vi "Double Acq test RT.vi"() -> ()   [LabVIEW 2014]
uses:
  <vilib>/Platform/TimedLoop/XDataNode/timing_clust.ctl
  <vilib>/Platform/TimedLoop/XDataNode/nitl_modes.ctl
  <vilib>/Platform/TimedLoop/XDataNode/wakeup.ctl
  <vilib>/FPGAPlugInAG/sbRIO-9636/niLvFpga_Open_sbRIO-9636.vi
  <vilib>/rvi/interface/common/dynamic/niFpgaDynamicAddResources.vi
  <vilib>/rvi/interface/common/niFpgaWaitOnOcc.vi
  <vilib>/Utility/error.llb/Error Cluster From Error Code.vi
  <vilib>/FPGAPlugInAG/Dynamic/niLvFpga_Run_Dynamic.vi
  <vilib>/rvi/errors/niLvFpgaAdjustHostInterfaceError.vi
  <vilib>/FPGAPlugInAG/Dynamic/niLvFpga_Abort_Dynamic.vi
  <vilib>/FPGAPlugInAG/Dynamic/niLvFpga_Close_Dynamic.vi
  <vilib>/rvi/interface/nirviOpenFPGA/nirviOpenFPGA.xnode
  FPGA Bitfiles/LaserDistanceSen_FPGATarget_DoubleAcquisitio_6KO4bY+0XGM.lvbitx
  FPGA Target/Test VIs/Double Acquisition (Mod-Sign) test.vi
  <vilib>/rvi/interface/nirviMethod/nirviMethod.xnode
  <vilib>/Platform/TimedLoop/XDataNode/XDataNode.xnode
  <vilib>/rvi/interface/nirviReadWriteControl/nirviReadWriteControl.xnode
  <vilib>/rvi/interface/nirviCloseFPGA/nirviCloseFPGA.xnode
  <vilib>/rvi/interface/Simulation/niFpgaSimulationCallBeginRW.vi
  <vilib>/FPGAPlugInAG/Dynamic/niLvFpga_ConfigureFifo_Dynamic.vi
  <vilib>/rvi/errors/niLvFpgaMergeErrorWithErrorCode.vi
  <vilib>/FPGAPlugInAG/Dynamic/niLvFpga_StartFifo_Dynamic.vi
  <vilib>/FPGAPlugInAG/Dynamic/niLvFpga_ReadFifo_Dynamic.vi
  <vilib>/Platform/TimedLoop/XDataNode/XDNodeRunTimeDep.lvlib
  NiFpgaLv.dll
panel:
  out "Modulation Signal":dbl[](graph)
  out "Signal":dbl[](graph)
  in  "stop":bool
  in  "Snapshot":bool
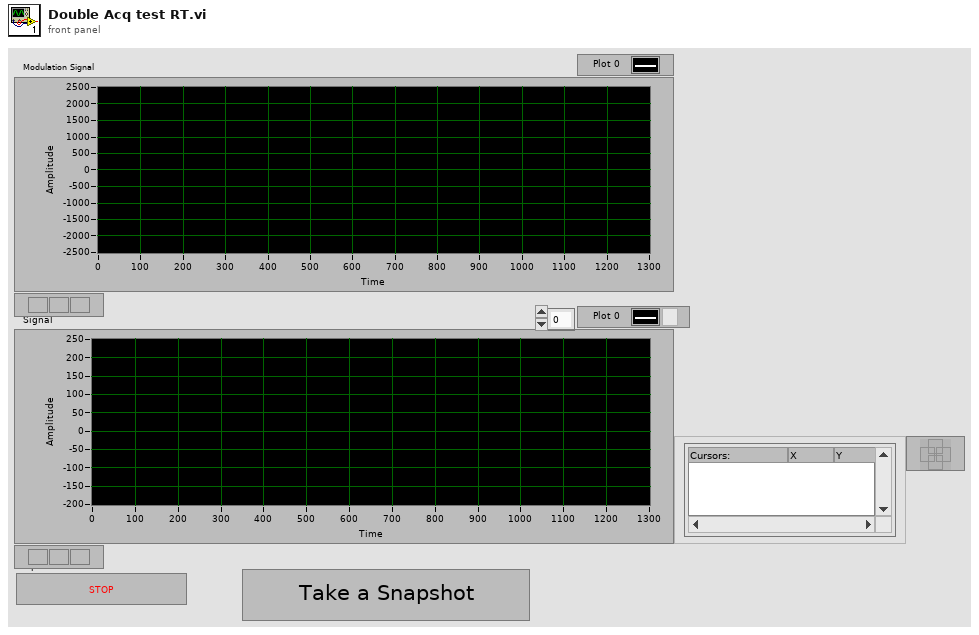
[diagram p1: front panel]
types:
  T1 = typedef "XDNodeRunTimeDep.lvlib/timing_clust.ctl" = cluster{"Expected End [f-1]":u64, "Actual End [f-1]":u64, "Finished Late? [f-1]":bool, "Expected End [i-1]":u64, "Actual End [i-1]":u64, "Finished Late? [i-1]":bool, "Expected Start [i]":u64, "Actual Start [i]":u64, "Expected Start [f]":u64, "Actual Start [f]":u64, "Source Name":string, "Structure Name":string, "Period":i64, "Deadline":i64, "Offset":i64, "Start":i64, "Priority":i32, "Timeout":i32, "Mode":T2, "Wakeup Reason":T3, "Error":errorcluster, "Source Type":string, "Secondary Source Type":string, "Global End Time":u64, "Global Start Time":u64, "Frame Duration":u64, "Iteration Duration":u64, "Assigned CPU":i32, "I/O Scan Engine Mode":u32}
  T2 = typedef "XDNodeRunTimeDep.lvlib/nitl_modes.ctl" = enum32{"No Change", "Process missed periods, maintain original phase", "Discard missed periods, maintain original phase", "Process missed periods, ignore original phase", "Discard missed periods, ignore original phase"}
  T3 = typedef "XDNodeRunTimeDep.lvlib/wakeup.ctl" = enum32{"Normal", "Aborted", "Asynchronous wakeup", "Timing source error", "Timed loop error", "Timeout"}
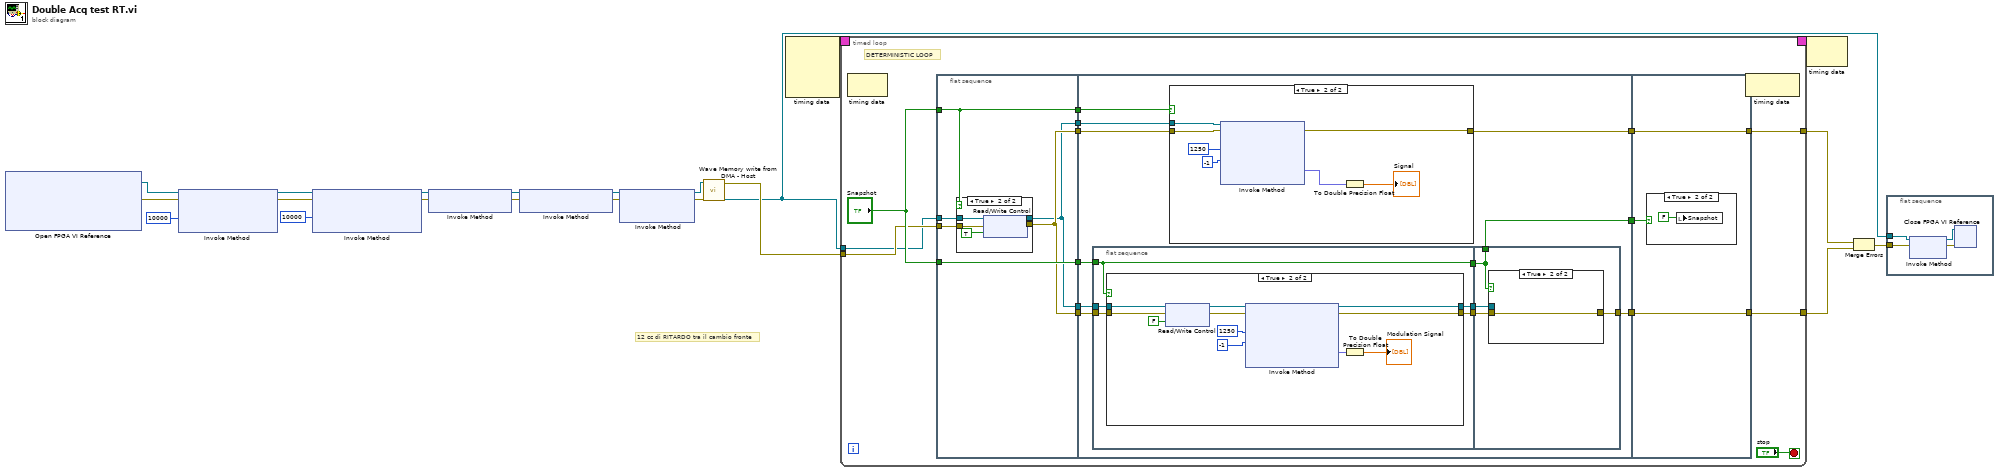
[diagram p0: block diagram]
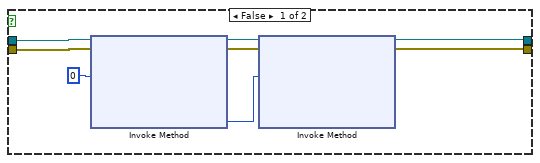
[diagram p3: hidden frame]
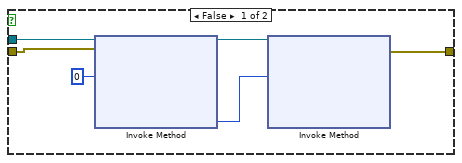
[diagram p5: hidden frame]
diagram:
  # "12 cc di RITARDO tra il cambio fronte"
  n1 = xnode "Open FPGA VI Reference"() -> ("FPGA VI Reference Out"=w8:refnum<k20>, "error out"=w9:errorcluster)  [unwired: 2 in]
  n2 = xnode "Invoke Method"("FPGA VI Reference In"=w8, "error in"=w9, "Requested Depth"=u32 10000) -> ("FPGA VI Reference Out"=w19:refnum<k20>, "error out"=w18:errorcluster)  [unwired: 1 out]
  n3 = xnode "Invoke Method"("FPGA VI Reference In"=w19, "error in"=w18, "Requested Depth"=u32 10000) -> ("FPGA VI Reference Out"=w6:refnum<k20>, "error out"=w7:errorcluster)  [unwired: 1 out]
  n4 = xnode "Invoke Method"("FPGA VI Reference In"=w6, "error in"=w7) -> ("FPGA VI Reference Out"=w15:refnum<k20>, "error out"=w14:errorcluster)
  n5 = xnode "Invoke Method"("FPGA VI Reference In"=w15, "error in"=w14) -> ("FPGA VI Reference Out"=w4:refnum<k20>, "error out"=w5:errorcluster)
  n6 = xnode "Invoke Method"("FPGA VI Reference In"=w4, "error in"=w5) -> ("FPGA VI Reference Out"=w12:refnum<k20>, "error out"=w11:errorcluster)  [unwired: 1 in]
  n7 = call "Wave Memory write from DMA - Host.vi"("error in"=w11, "FPGA VI Reference In"=w12) -> ("FPGA VI Reference Out"=w1:refnum<k20>, "error out"=w3:errorcluster)  [unwired: 7 in, 1 out]
  n8 = node-c288() -> (w21:T1)  [unwired: 4 in]
  n9 = timed-loop {
    tunnel: w1 -> [w32]
    tunnel: w3 -> [w33]
    tunnel: [w35] -> w2
    tunnel: [w36] -> w10
    timing: w21 -> [_]
    timing-out: [_] -> w20
    stop <- "stop" stop-if-true
    # "DETERMINISTIC LOOP"
    n10 = node-c288() -> ()  [unwired: 1 in, 1 out]
    n11 = flat-sequence {
      tunnel: w32 -> [w41]
      tunnel: w33 -> [w42]
      tunnel: "Snapshot" -> [w39]
      tunnel: "Snapshot" -> [w44]
      tunnel: [w43] -> w31
      tunnel: [w44] -> w30
      tunnel: [w39] -> w29
      tunnel: [w43] -> w28
      tunnel: [w40] -> w27
      tunnel: [w40] -> w26
      tunnel: w31 -> [w59]
      tunnel: w30 -> [w52]
      tunnel: w29 -> [w56]
      tunnel: w28 -> [w55]
      tunnel: w27 -> [w54]
      tunnel: w26 -> [w60]
      tunnel: [w58] -> w25
      tunnel: [w57] -> w24
      tunnel: [w53] -> w23
      tunnel: [w108] -> w35
      tunnel: [w109] -> w36
      tunnel: w25 -> [w109]
      tunnel: w24 -> [w108]
      tunnel: w23 -> [w107]
      frame #0 {
        n12 = case shown="True" w39 {
          tunnel: [w45 w50] -> w43
          tunnel: w42 -> [w45 w49]
          tunnel: w41 -> [w46 w48]
          tunnel: [w46 w47] -> w40
          frame False {
          }
          frame True {
            n13 = xnode "Read/Write Control"("FPGA VI Reference In"=w48, "error in"=w49, "Snapshot"=TRUE ("snapshot")) -> ("FPGA VI Reference Out"=w47:refnum<k20>, "error out"=w50:errorcluster)
          }
        }
      }
      frame #1 {
        n14 = flat-sequence {
          tunnel: w60 -> [w68]
          tunnel: w59 -> [w67]
          tunnel: w52 -> [w64]
          tunnel: [w66] -> w63
          tunnel: [w65] -> w62
          tunnel: [w64] -> w61
          tunnel: [w89] -> w57
          tunnel: w63 -> [w91]
          tunnel: w62 -> [w90]
          tunnel: w61 -> [w88]
          tunnel: [w88] -> w53
          frame #0 {
            n15 = case shown="True" w64 {
              tunnel: w68 -> [w75 w78]
              tunnel: w67 -> [w73 w80]
              tunnel: [w72 w85] -> w65
              tunnel: [w69 w84] -> w66
              frame False {
                n16 = xnode "Invoke Method"("FPGA VI Reference In"=w75, "error in"=w73, "Number of Elements"=u32 0) -> ("FPGA VI Reference Out"=w71:refnum<k20>, "error out"=w70:errorcluster, "Elements Remaining"=w74:u32)  [unwired: 1 in, 1 out]
                n17 = xnode "Invoke Method"("FPGA VI Reference In"=w71, "error in"=w70, "Number of Elements"=w74) -> ("FPGA VI Reference Out"=w69:refnum<k20>, "error out"=w72:errorcluster)  [unwired: 1 in, 2 out]
              }
              frame True {
                n18 = xnode "Read/Write Control"("FPGA VI Reference In"=w78, "error in"=w80, "Snapshot"=FALSE ("snapshot")) -> ("FPGA VI Reference Out"=w77:refnum<k20>, "error out"=w79:errorcluster)
                n19 = xnode "Invoke Method"("FPGA VI Reference In"=w77, "error in"=w79, "Number of Elements"=u32 1250, "Timeout (ms)"=-1) -> ("FPGA VI Reference Out"=w84:refnum<k20>, "error out"=w85:errorcluster, "Data"=w83:fxp<+/-,12,12>[])  [unwired: 1 out]
                n20 = To Double Precision Float(number=w83) -> (double precision float=→"Modulation Signal":dbl[])
              }
            }
          }
          frame #1 {
            n21 = case shown="True" w88 {
              tunnel: [w92 w93] -> w89
              tunnel: w91 -> [_ _]
              tunnel: w90 -> [w92 w93]
              frame False {
              }
              frame True {
              }
            }
          }
        }
        n22 = case shown="True" w56 {
          tunnel: w54 -> [w98 w102]
          tunnel: w55 -> [w95 w103]
          tunnel: [w94 w106] -> w58
          frame False {
            n23 = xnode "Invoke Method"("FPGA VI Reference In"=w98, "error in"=w95, "Number of Elements"=u32 0) -> ("FPGA VI Reference Out"=w96:refnum<k20>, "Elements Remaining"=w97:u32)  [unwired: 1 in, 2 out]
            n24 = xnode "Invoke Method"("FPGA VI Reference In"=w96, "Number of Elements"=w97) -> ("error out"=w94:errorcluster)  [unwired: 2 in, 3 out]
          }
          frame True {
            n25 = xnode "Invoke Method"("FPGA VI Reference In"=w102, "error in"=w103, "Number of Elements"=u32 1250, "Timeout (ms)"=-1) -> ("error out"=w106:errorcluster, "Data"=w101:fxp<+/-,12,12>[])  [unwired: 2 out]
            n26 = To Double Precision Float(number=w101) -> (double precision float=→"Signal":dbl[])
          }
        }
      }
      frame #2 {
        n27 = case shown="True" w107 {
          frame False {
          }
          frame True {
            n28 = local write "Snapshot"(FALSE ("Snapshot")) -> ()
          }
        }
      }
    }
    n29 = node-c288() -> ()  [unwired: 1 in, 1 out]
  }
  n30 = node-c288(w20) -> ()  [unwired: 1 out]
  n31 = Merge Errors(w10, w2) -> (w13:errorcluster)
  n32 = flat-sequence {
    tunnel: w13 -> [w112]
    tunnel: w1 -> [w111]
    frame #0 {
      n33 = xnode "Invoke Method"("FPGA VI Reference In"=w111, "error in"=w112) -> ("FPGA VI Reference Out"=w113:refnum<k20>, "error out"=w114:errorcluster)
      n34 = xnode "Close FPGA VI Reference"("FPGA VI Reference In"=w113, "error in"=w114) -> ()  [unwired: 1 out]
    }
  }
